vi "Configure Measurement (Setup and Hold).vi"(0 "VISA resource name":refnum<visa-resource-name>, 1 "Clock Source (2: Channel 2)":i32(ring)=2 items=["Channel 1"=1, "Channel 2"=2, "Channel 3"=3, "Channel 4"=4, "Function 1"=5, "Function 2"=6, "Function 3"=7, "Function 4"=8, "Memory 1"=9, "Memory 2"=10, "Memory 3"=11, "Memory 4"=12, "Clock"=15, "MTrend"=16, "MSpectrum"=17, "Equalized"=18, "DIG 0"=20, "DIG 1"=21, "DIG 2"=22, "DIG 3"=23, "DIG 4"=24, "DIG 5"=25, "DIG 6"=26, "DIG 7"=27, "DIG 8"=28, "DIG 9"=29, "DIG 10"=30, "DIG 11"=31, "DIG 12"=32, "DIG 13"=33, "DIG 14"=34, "DIG 15"=35], 2 "Clock Source Direction (0: Rising)":i32(ring) items=["Rising", "Falling", "Both"], 5 "Data Source (1: Channel 1)":i32(ring)=1 items=["Channel 1"=1, "Channel 2"=2, "Channel 3"=3, "Channel 4"=4, "Function 1"=5, "Function 2"=6, "Function 3"=7, "Function 4"=8, "Memory 1"=9, "Memory 2"=10, "Memory 3"=11, "Memory 4"=12, "Clock"=15, "MTrend"=16, "MSpectrum"=17, "Equalized"=18], 7 "Data Source Direction (0: Rising)":i32(ring) items=["Rising", "Falling", "Both"], 9 "Measurement Function (0: Setup Time)":i32(ring) items=["Setup Time", "Hold Time"], 11 "error in (no error)":errorcluster) -> (4 "VISA resource name out":refnum<visa-resource-name>, 15 "error out":errorcluster)   [LabVIEW 2020, in "Agilent 90000 Series.lvlib"]
doc: "Configures the setup time/hold time measurement.\n\n<B>Note:</B>\nCalling this VI disables all previously enabled measurements and clears existing measurement results from display."
uses:
  Agilent 90000 Series.lvlib
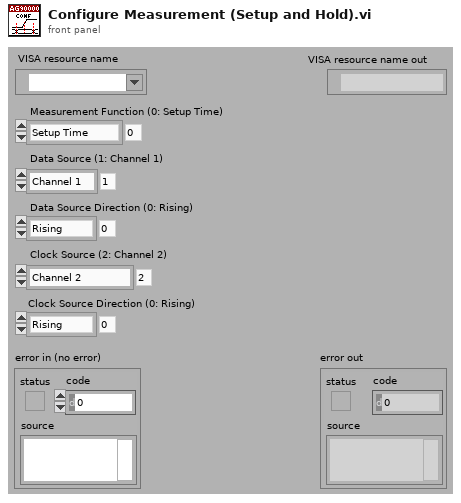
[diagram p1: front panel]
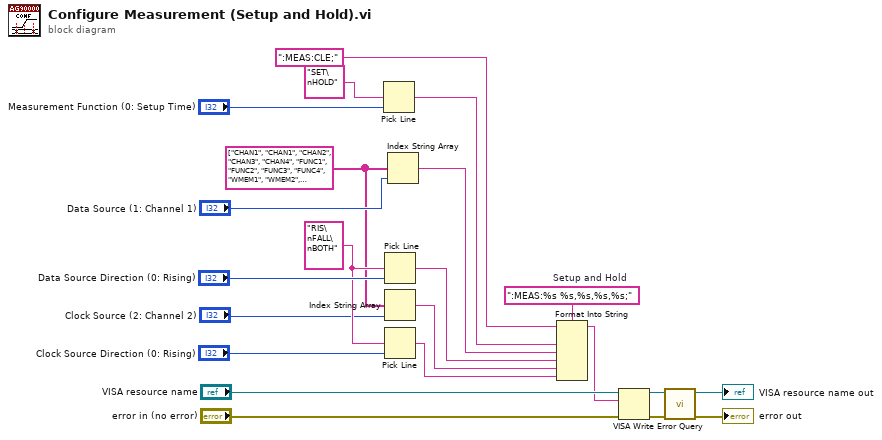
[diagram p0: block diagram]
diagram:
  w1 = string[] ["CHAN1", "CHAN1", "CHAN2", "CHAN3", "CHAN4", "FUNC1", "FUNC2", "FUNC3", "FUNC4", "WMEM1", "WMEM2", "WMEM3", "WMEM4", "AUX", "LINE", "CLOC", "MTR", "MSP", "EQU", "NONE", "DIG0", "DIG1", "DIG2", "DIG3", "DIG4", "DIG5", "DIG6", "DIG7", "DIG8", "DIG9", "DIG10", "DIG11", "DIG12", "DIG13", "DIG14", "DIG15", "", "", "", "", "", "POD1", "POD2", "", "", "", "", "", "", "", "", "BUS1", "BUS2", "BUS3", "BUS4", "", "", "", "", "", "", "DIFF1", "DIFF2", "", "", "", "", "", "", "", "", "COMM3", "COMM4"]
  w11 = ":MEAS:%s %s,%s,%s,%s;"  # Setup and Hold
  w12 = "RIS\nFALL\nBOTH" ("multi-line string")
  n1 = Pick Line(multi-line string="SET\nHOLD", line index="Measurement Function (0: Setup Time)") -> (output string=w10:string)  [unwired: 1 out]
  n2 = Pick Line(multi-line string=w12, line index="Data Source Direction (0: Rising)") -> (output string=w8:string)  [unwired: 1 out]
  n3 = Index String Array(1:"Clock Source (2: Channel 2)", 2:w1) -> (0:w7:string)  [unwired: 1 out]
  n4 = Pick Line(multi-line string=w12, line index="Clock Source Direction (0: Rising)") -> (output string=w6:string)  [unwired: 1 out]
  n5 = Index String Array(1:"Data Source (1: Channel 1)", 2:w1) -> (0:w9:string)  [unwired: 1 out]
  n6 = Format Into String(format string=w11, initial string=":MEAS:CLE;", w10, w9, w8, w7, w6) -> (resulting string=w4:string)  [unwired: 1 in, 1 out]
  n7 = VISA Write(VISA resource name="VISA resource name", write buffer=w4, error in (no error)="error in (no error)") -> (VISA resource name out=w18:refnum<visa-resource-name>, error out=w17:errorcluster)  [unwired: 1 out]
  n8 = call "Error Query.vi"("error in (no error)"=w17, "VISA resource name"=w18) -> ("error out"=→"error out":errorcluster, "VISA resource name out"=→"VISA resource name out":refnum<visa-resource-name>)  [unwired: 8 out]
